vi "trace_properties_double.vi"(0 "reference in":refnum<class "OSA.lvclass">, 2 "property":T3, 3 "dataType":T2, 4 "trace idx":u32, 5 "error in (no error)":errorcluster) -> (14 "reference out":refnum<class "OSA.lvclass">, 16 "property out":cluster{"property":string, "property value":dbl}, 17 "property out array":T1(array[cluster]), 19 "error out":errorcluster)   [LabVIEW 2010, in "OSA.lvclass"]
doc: "Trace properties returned as double."
uses:
  OSA.lvclass
  typeDef/trace_properties_double.ctl
  typeDef/acq_dataType.ctl
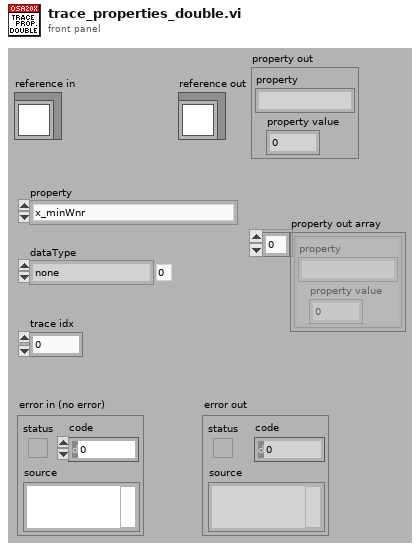
[diagram p1: front panel]
types:
  T1 = cluster{"property":string, "property value":dbl}[]
  T2 = typedef "OSA.lvclass/acq_dataType.ctl" = enum16{"none", "interferogram", "spectrum"}
  T3 = typedef "OSA.lvclass/trace_properties_double.ctl" = enum16{"x_minWnr", "x_maxWnr", "x_min", "x_max", "y_min", "y_max", "resolution", "referenceWavelength_nm_vac", "samplingDistance_cm_vac", "zeroFillFactor", "air_temp", "air_press", "air_relHum", "minOPD_cm", "maxOPD_cm", "interferogramOffset", "apodizationPowerCompensation", "integrationTime_ms", "gainLevel", "all_doubleProperties"}
  T4 = typedef "OSA.lvclass/ObjectAttributes.ctl" = cluster{"Stop":bool, "dataType":T2, "spectrometerIdx":u16, "buffer size interferogram":i32, "interferogram":cluster{"new":bool, "plot_x_ min":sgl, "plot_x_max":sgl, "plot_y_min":sgl, "plot_y_max":sgl, "Graph Intrfrgrm":T5, "timeStamp":u32, "signal (%)":dbl, "traces":cluster{"idx":u32, "broadBand":bool, "monoChromatic":bool, "peakToPeakSignal":dbl, "peakToPeakPos":dbl}[], "traces idx last":i32}, "spectrum":cluster{"new":bool, "plot_x_min":sgl, "plot_x_max":sgl, "plot_unit_x":T6, "plot_unit_y":T7, "plot_y_min":sgl, "plot_y_max":sgl, "Graph Spectrum":T5, "timeStamp":u32, "X_VAL_OPTIONS":enum16{"MIN_MAX", "ARRAY"}, "traces":cluster{"idx":u32}[], "traces idx last":i32}, "Thorlabs_OSA_64.lvclass:queue_action.ctlqueue ref":refnum<queue>, "action":T8, "plot zoom step":dbl, "buffer semaphore":T9, "acq stopped":bool, "dataType active":T2, "temperature (degr C)":sgl, "pressure (hPa)":sgl, "rel humidity (%)":sgl, "settings":cluster{"resolution":T10, "sensitivity":T11, "Average":bool, "average nr":u32, "apodisation":T12, "acq delay (ms)":u32, "airMesure":T13, "wmtr on":bool, "intfgrm_smooth_width":u16, "intfgrm_smooth_nrOfPasses":u16, "intfgrm_smooth":T14, "phaseCorrection":T15, "zeroFill":u8, "spectr_smooth":T14, "spectr_smooth_width":u16, "spectr_smooth_nrOfPasses":u16, "resolution (/cm)":sgl, "REF wavelength, (nm)":dbl, "gain_idx":u16, "gainAuto":bool, "gain_relative":dbl, "PD sensitivity mode":T16, "PD senseMode implemented":bool, "SensorTemperature implemented":bool, "SensorPressure implemented":bool, "SensorHumidity implemented":bool}, "peaks position":sgl[], "peaks width":sgl[], "peaks height":sgl[], "peaks max nr":u32, "peaks latest nr":i32, "peaks new":bool, "power":dbl, "power new":bool, "path":string, "wavelength (WNr)":dbl, "wavelength new":bool, "buffer size spectrum":i32, "status":string, "VI reference":refnum<vi>, "funcPointer":u64, "libraryPointer":u64, "singleAcquisition":bool, "coherenceLength (cm)":dbl, "coherenceLength new":bool, "spectrometer model":string, "spectrometer serial nr":string, "peaks thld left":sgl[], "peaks thld right":sgl[], "coherenceLength error (cm)":dbl, "ADC bits":u16, "peaks position centroid":sgl[], "peaks height centroid":sgl[], "OSA series":T17, "channel":u16, "channels_nr":i32, "channel stiched":u32, "channelType_spectrum":T18}
  T5 = typedef "OSA.lvclass/graph_intensity.ctl" = refnum<vi>
  T6 = typedef "OSA.lvclass/spectrum_x_unit.ctl" = enum16{"wavenr/cm", "THz", "eV", "nm_air", "nm_vac"}
  T7 = typedef "OSA.lvclass/y_unit.ctl" = enum16{"ADC counts", "dBm pwr absolute", "dBm pwr density", "mW pwr absolute", "mW pwr density"}
  T8 = typedef "OSA.lvclass/queue_action.ctl" = enum16{"none", "stop", "GUI_plotInterferogram", "GUI_plotSpectrum", "GUI_plotInterferogramRescale", "GUI_plotSpectrumRescale", "GUI_plotInterferogramReset", "GUI_plotSpectrumReset", "GUI_plotInterferogramAutoScaleY", "GUI_plotSpectrumAutoScaleY", "GUI_plotInterferogramZoomOut", "GUI_plotSpectrumZoomOut", "GUI_plotInterferogramPane", "GUI_plotSpectrumPane", "GUI_plotInterferogramZoomMouse", "GUI_plotSpectrumZoomMouse", "ENVIRONMENT temperature", "ENVIRONMENT pressure", "MODE_resolution set", "MODE_resolution get", "MODE_sensitivity set", "MODE_sensitivity get", "MODE_PDTemperature set", "MODE_PDTemperature get", "REBOOT/RESET firmware", "ACQASYNC_acquireSingleSpectrum", "ACQASYNC_continuous start", "ACQASYNC_continuous stop\n", "ACQASYNC_get last interferogram", "ACQASYNC_get last spectrum", "ACQASYNC_get last waveNr", "ACQOPT_interferogram smoothing set", "ACQOPT_interferogram smoothing get", "ACQOPT_spectrum smoothing set", "ACQOPT_spectrum smoothing get", "ACQOPT_apodisation type set", "ACQOPT_apodisation type get", "ACQOPT_phase correction type set", "ACQOPT_phase correction type get", "ACQOPT_acqIntervall_set", "ACQOPT_acqIntervall_get", "ACQOPT_average spectrum set", "ACQOPT_average spectrum get", "ACQOPT_rolling average set", "ACQOPT_rolling average get", "ACQOPT_zero fill factor set", "ACQOPT_zero fill factor get", "ACQOPT_cycle counting set", "ACQOPT_cycle counting get", "ACQOPT_air measure option set", "ACQOPT_air measure option get", "ACQOPT_gainLevel auto get", "ACQOPT_gainLevel auto set", "ACQOPT_gainLevel get", "ACQOPT_gainLevel set", "ACQOPT_getAll", "INSTRUMENT_PROPERTY_range_WaveNr_min", "INSTRUMENT_PROPERTY_range_WaveNr_max", "INSTRUMENT_PROPERTY_reference_wavelength_cm^-1", "INSTRUMENT_PROPERTY_samplesPerRefPeriod", "INSTRUMENT_PROPERTY_resolution_waveNrPercm", "INSTRUMENT_PROPERTY_availableGainLevels", "INSTRUMENT_PROPERTY_status", "CONVERT", "ANALYSE_POWER", "ANALYSE_PEAKS", "ANALYSE_WAVELENGTH", "ANALYSE_SPECTRUM", "ANALYSE_INTERFEROGRAM", "ANALYSE_COHERENCE_LENGTH", "MATH", "MATH_power", "MATH_peaks", "FILE", "miscellaneous"}
  T9 = typedef "Semaphore RefNum" = refnum<k1>
  T10 = typedef "OSA.lvclass/resolution.ctl" = enum16{"low", "high"}
  T11 = typedef "OSA.lvclass/sensitivityMode.ctl" = enum16{"low", "low medium", "high medium", "high"}
  T12 = typedef "OSA.lvclass/apodisation.ctl" = enum16{"NONE", "NORTON_BEER_WEAK", "NORTON_BEER_MEDIUM", "NORTON_BEER_STRONG", "TRIANGULAR", "COSINE", "HANN", "HAMMING", "BLACKMANHARRIS3", "BLACKMANHARRIS4", "GAUSSIAN"}
  T13 = typedef "OSA.lvclass/airMeasure.ctl" = enum16{"TEMPERATURE", "PRESSURE"}
  T14 = typedef "OSA.lvclass/smoothing.ctl" = enum16{"NONE", "BINOMIAL", "SAVITSKY_GOLAY", "FOURIER", "MOVING_AVERAGE", "GAUSSIAN"}
  T15 = typedef "OSA.lvclass/phaseCorrection.ctl" = enum16{"NONE", "MERTZ", "FORMAN", "MERTZ_FILE", "FORMAN_FILE", "FUTURE COMP."}
  T16 = typedef "OSA.lvclass/PDTemperatureMode.ctl" = enum16{"cool: better sensitivity/noise floor", "warm: extended wl range"}
  T17 = typedef "OSA_series.ctl" = enum16{"OSA200", "OSA300", "UNKNOWN"}
  T18 = typedef "OSA.lvclass/channelType_spectrum.ctl" = enum16{"SINGLE CHANNEL", "STICHED"}
  T19 = cluster{"idx":u32, "broadBand":bool, "monoChromatic":bool, "peakToPeakSignal":dbl, "peakToPeakPos":dbl}[]
  T20 = enum16{"x_minWnr", "x_maxWnr", "x_min", "x_max", "y_min", "y_max", "resolution", "referenceWavelength_nm_vac", "samplingDistance_cm_vac", "zeroFillFactor", "air_temp", "air_press", "air_relHum", "minOPD_cm", "maxOPD_cm", "interferogramOffset", "apodizationPowerCompensation", "integrationTime_ms", "gainLevel", "all_doubleProperties"}
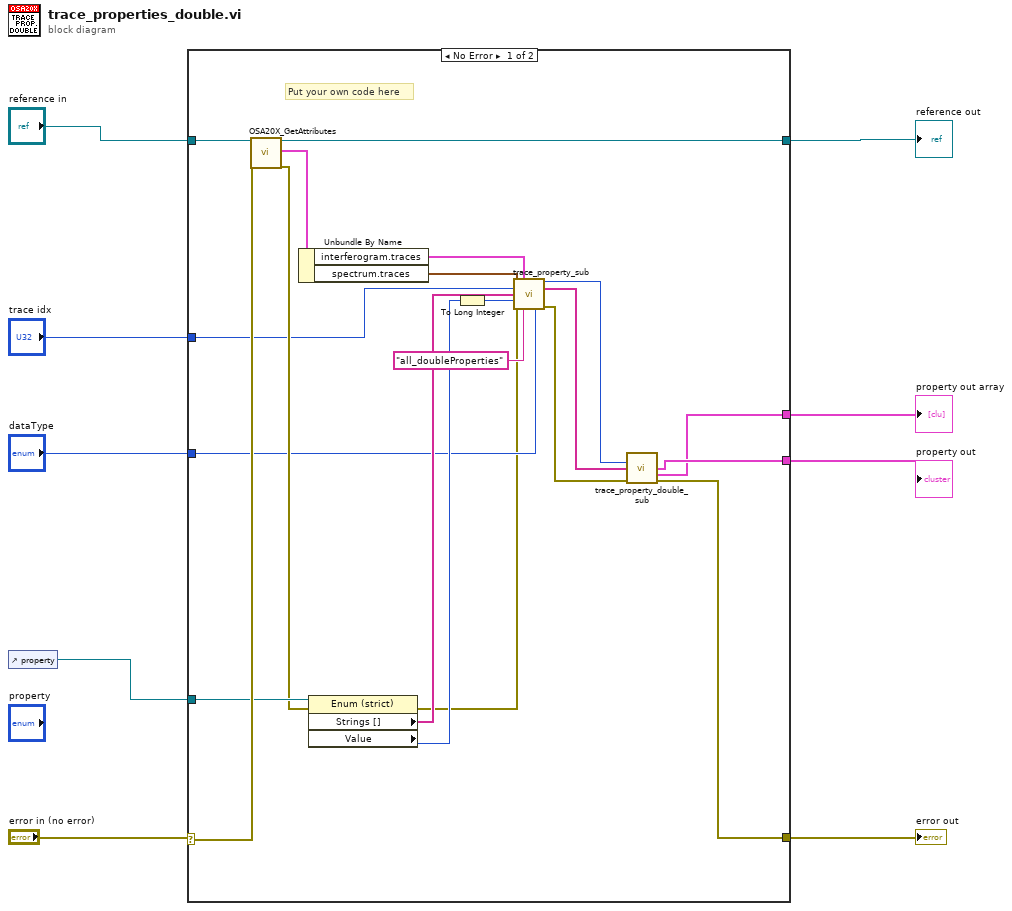
[diagram p0: block diagram]
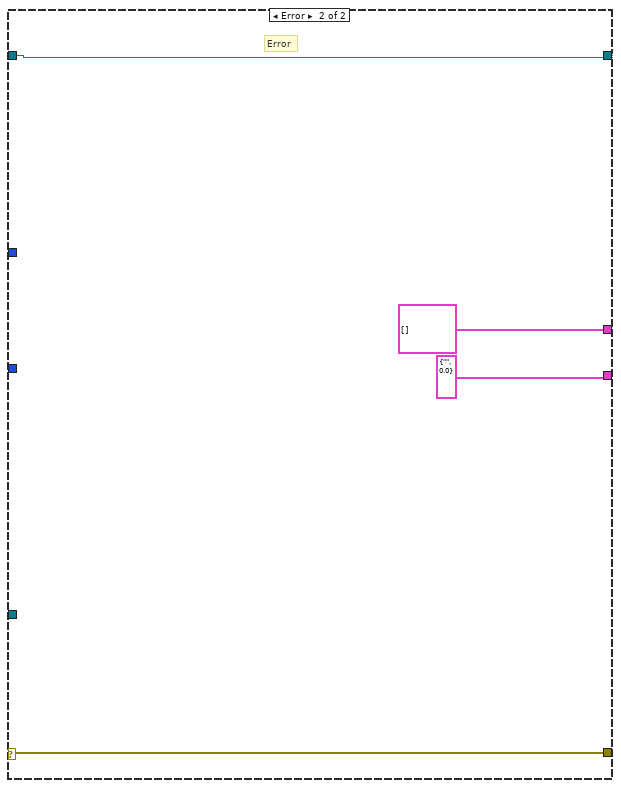
[diagram p2: hidden frame]
diagram:
  n1 = control-ref of="property"() -> (w4:refnum<vi>)
  n2 = case shown="No Error" "error in (no error)" {
    selector: "error in (no error)" -> [w29 w34]
    tunnel: [w12 w34] -> w9
    tunnel: "reference in" -> [w28 w33]
    tunnel: [w27 w33] -> w1
    tunnel: "dataType" -> [w19 _]
    tunnel: "trace idx" -> [w22 _]
    tunnel: w4 -> [w26 _]
    tunnel: [w11 cluster{"property":string, "property value":dbl} {"property"="", "property value"=0.0}] -> w2
    tunnel: [w10 T1 []] -> w3
    frame No Error {
      # "Put your own code here"
      n3 = call "OSA20X_GetAttributes.vi"("reference in"=w28, "error in (no error)"=w29) -> ("reference out"=w27:refnum<class "OSA.lvclass">, "Data"=w30:T4, "error out"=w25:errorcluster)  [unwired: 14 in, 1 out]
      n4 = Unbundle By Name(w30) -> ("interferogram.traces"=w24:T19, "spectrum.traces"=w23:cluster{"idx":u32}[])
      n5 = property class="Enum (strict)"(reference=w26, error in=w25) -> (error out=w16:errorcluster, "Strings []"=w21:string[], "Value"=w20:T20)  [unwired: 1 out]
      n6 = To Long Integer(number=w20) -> (32bit integer=w17:i32)
      n7 = call "trace_property_sub.vi"("traces_spectrum"=w23, "traces_interferogram"=w24, "trace idx"=w22, "Strings enum"=w21, "Value enum"=w17, "error in (no error)"=w16, "all string"="all_doubleProperties", "dataType"=w19) -> ("global trace idx"=w15:u32, "parameter names"=w14:string[], "error out"=w13:errorcluster)  [unwired: 4 in, 1 out]
      n8 = call "trace_property_double_sub.vi"("trace idx global"=w15, "properties ui"=w14, "error in (no error)"=w13) -> ("property"=w11:cluster{"property":string, "property value":dbl}, "properties"=w10:T1, "error out"=w12:errorcluster)  [unwired: 10 in]
    }
    frame Error {
      # "Error"
    }
  }
  "error out" <- w9
  "reference out" <- w1
  "property out array" <- w3
  "property out" <- w2
